vi "REPORT_OPRTN_reshape_records_for_display.vi"(11 "records_from_SQL":string[][](array[string])) -> (3 "records_to_display":string[][](array[string]), 4 "archivisation_description":string[][](array[string]), 5 "column_headers":string[](array[string]), 7 "number_of_static_columns":i32=4)   [LabVIEW 2019]
uses:
  _misc/AULocalize/SubVIs/Get Localized Phrase Compact Interface 1D.vi
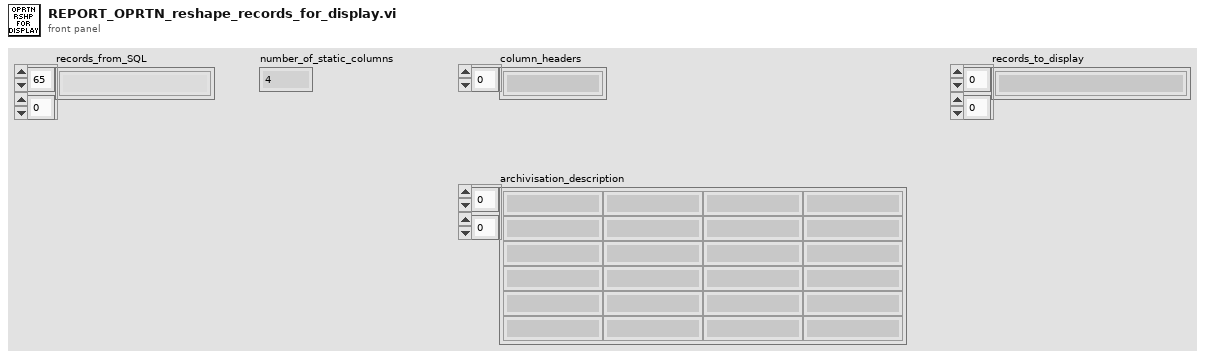
[diagram p1: front panel]
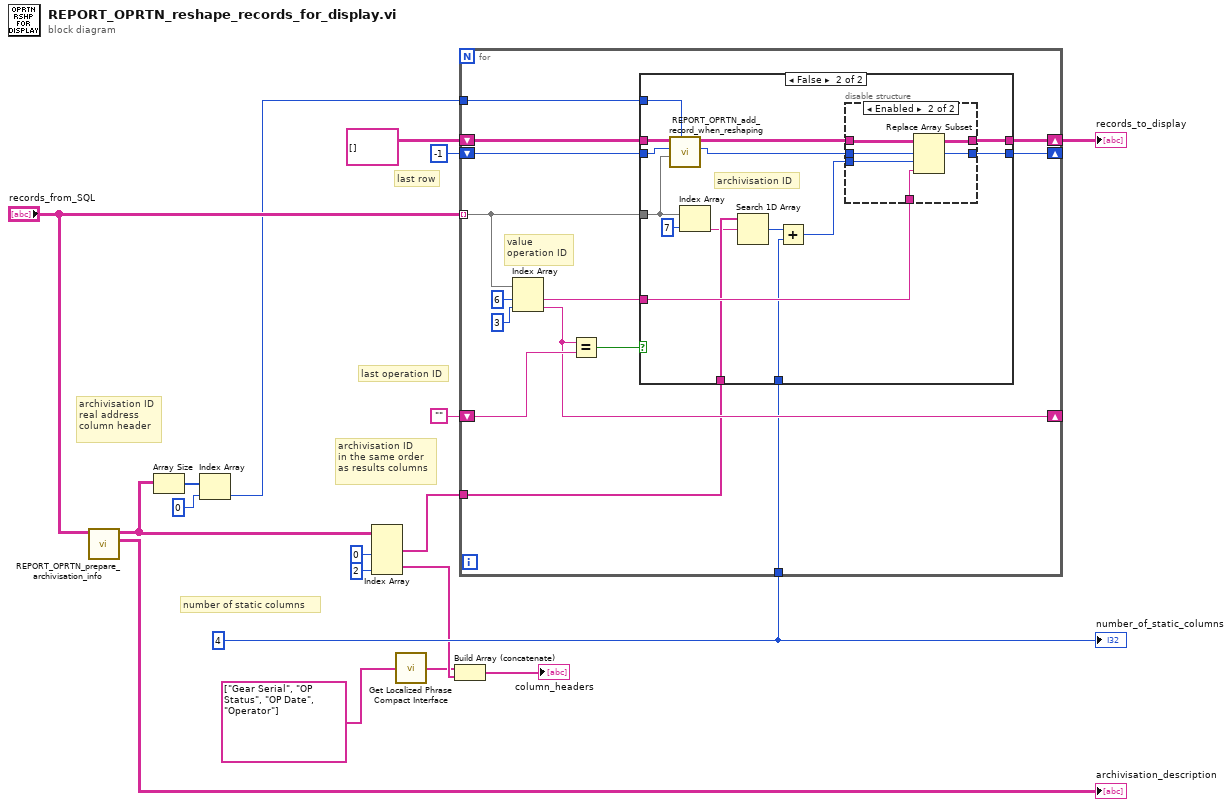
[diagram p0: block diagram]
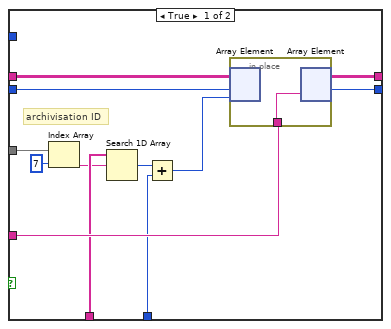
[diagram p2: hidden frame]
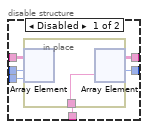
[diagram p3: hidden frame]
diagram:
  w9 = 4 ("x")
  # "number of static columns"
  # "archivisation ID\nin the same order\nas results columns"
  # "last row"
  # "archivisation ID\nreal address\ncolumn header"
  # "last operation ID"
  n1 = call "REPORT_OPRTN_prepare_archivisation_info.vi"("records_from_SQL"="records_from_SQL") -> ("archivisation_description"=→"archivisation_description":string[][], "archivisation_info"=w12:string[][])  [unwired: 9 in]
  n2 = Array Size(array=w12) -> (size(s)=w15:i32[])
  n3 = Index Array(array=w15, index=0) -> (element=w4:i32)
  n4 = Index Array(array=w12, index (col) #1=0 ("disabled index (col)"), index (col) #2=2 ("index (col)")) -> (element #1=w10:string[], element #2=w6:string[])  [unwired: 2 in]
  n5 = call-poly "Get Localized Phrase Compact Interface.vi"("Key"=string[] ["Gear Serial", "OP Status", "OP Date", "Operator"]) -> ("Translated Phrase"=w1:string[])
  n6 = Build Array (concatenate)(w1, w6) -> (→"column_headers":string[])
  n7 = for {
    tunnel: "records_from_SQL" -> [w27] mode=indexing
    shift-right: [w30] -> _
    shift-left: "" -> [w31]
    shift-right: [w26] -> w17
    shift-left: string[][] [] -> [w28]
    shift-right: [w24] -> _
    shift-left: -1 ("index") -> [w25]
    tunnel: w10 -> [w22]
    tunnel: w9 -> [w21]
    tunnel: w4 -> [w19]
    # "value\noperation ID"
    n8 = Index Array(array=w27, index #1=6 ("index"), index #2=3 ("index")) -> (element #1=w20:string, element #2=w30:string)
    n9 = Equal?(x=w30, y=w31) -> (x = y?=w29:bool)
    n10 = case shown="False" w29 {
      tunnel: w28 -> [w44 w51]
      tunnel: w27 -> [w38 w47]
      tunnel: [w43 w60] -> w26
      tunnel: w25 -> [w42 w49]
      tunnel: [w40 w58] -> w24
      tunnel: w20 -> [w41 w59]
      tunnel: w22 -> [w39 w57]
      tunnel: w21 -> [w34 w53]
      tunnel: w19 -> [_ w46]
      frame True {
        # "archivisation ID"
        n11 = Index Array(array=w38, index=7) -> (element=w36:string)
        n12 = Search 1D Array(1D array=w39, element=w36) -> (index of element=w35:i32)  [unwired: 1 in]
        n13 = Add(x=w35, y=w34) -> (x+y=w33:i32)
        n14 = in-place {
          in-place-border: w41 -> [w45]
          n15 = in-place-array #1(w44, w42, w33) -> ()  [unwired: 1 out]
          n16 = in-place-array #1(w45) -> (w43:string[][], w40:i32)  [unwired: 1 out]
        }
      }
      frame False {
        # "archivisation ID"
        n17 = call "REPORT_OPRTN_add_record_when_reshaping.vi"("no_of_dynamic_columns"=w46, "records_from_SQL"=w47, "last_row_in"=w49, "records_to_display_in"=w51) -> ("last_row_out"=w48:i32, "records_to_display_out"=w50:string[][])  [unwired: 6 in]
        n18 = Index Array(array=w47, index=7) -> (element=w55:string)
        n19 = Search 1D Array(1D array=w57, element=w55) -> (index of element=w54:i32)  [unwired: 1 in]
        n20 = Add(x=w54, y=w53) -> (x+y=w52:i32)
        n21 = disable-structure shown="Enabled" {
          disable-tunnel: [w66 w71] -> w60
          disable-tunnel: w59 -> [w65 w69]
          disable-tunnel: [w64 w68] -> w58
          disable-tunnel: w52 -> [w63 w70]
          disable-tunnel: w50 -> [w62 w72]
          disable-tunnel: w48 -> [w61 w68]
          frame Disabled {
            n22 = in-place {
              in-place-border: w65 -> [w67]
              n23 = in-place-array #2(w62, w61, w63) -> ()  [unwired: 1 out]
              n24 = in-place-array #2(w67) -> (w66:string[][], w64:i32)  [unwired: 1 out]
            }
          }
          frame Enabled {
            n25 = Replace Array Subset(array=w72, new element=w69, index (row)=w68, index (col)=w70) -> (w71:string[][])
          }
        }
      }
    }
  }
  "records_to_display" <- w17
  "number_of_static_columns" <- w9
